vi "Double Array To Waveform.vi"(11 "Double Array Data":cluster{"double Array{X}":dbl[]}[](array[cluster])) -> (3 "Waveform Data":waveform(dbl)[](array[waveform]))   [LabVIEW 2017]
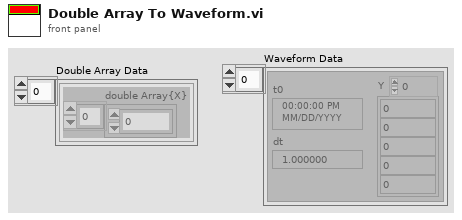
[diagram p1: front panel]
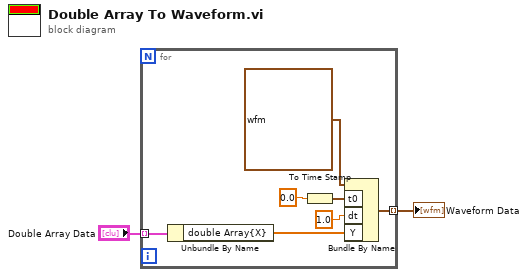
[diagram p0: block diagram]
diagram:
  n1 = for {
    tunnel: "Double Array Data" -> [w8] mode=indexing
    tunnel: [w7] -> w2 mode=indexing
    n2 = Unbundle By Name(w8) -> ("double Array{X}"=w6:dbl[])
    n3 = To Time Stamp(1:0.0 ("dt")) -> (0:w3:timestamp)
    n4 = Bundle By Name(cluster=waveform(dbl) {"t0"=timestamp(0 s since 1904-01-01), "dt"=1.0, "Y"=[]} ("Waveform"), "t0"=w3, "dt"=1.0, "Y"=w6) -> (w7:waveform(dbl))
  }
  "Waveform Data" <- w2
